vi "svl_Init Arrays for Exp Avg.vi"(0 "scaled signals":waveform(dbl)[](array[waveform]), 11 "error in (no error)":errorcluster) -> (4 "scaled signals":waveform(dbl)[](array[waveform]), 8 "initial values (impulse)":dbl[](array[numeric]) format="%.2f", 10 "dt":dbl, 14 "initial values (exp)":dbl[](array[numeric]) format="%.2f", 15 "error out":errorcluster)   [LabVIEW 2017]
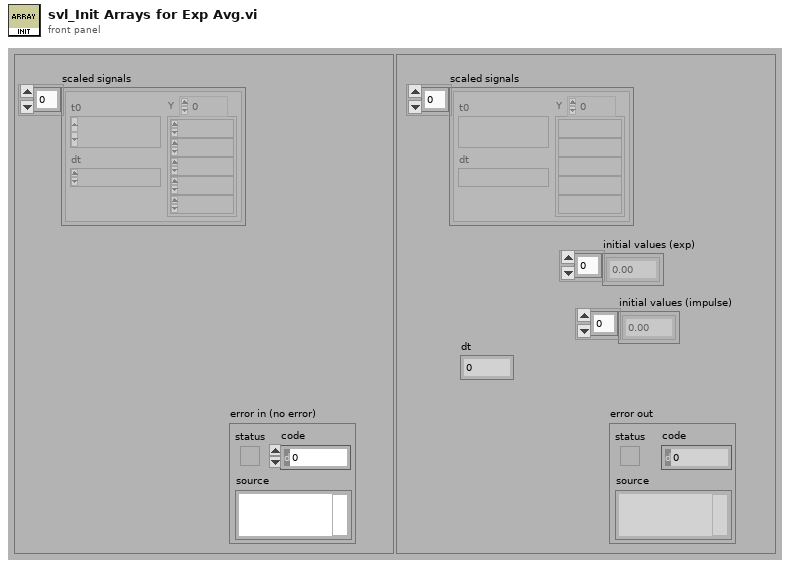
[diagram p1: front panel]
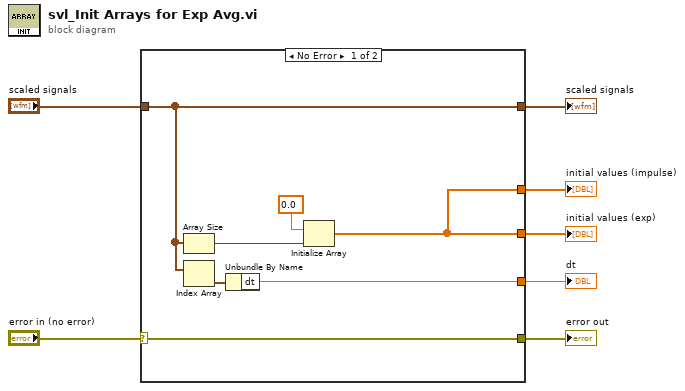
[diagram p0: block diagram]
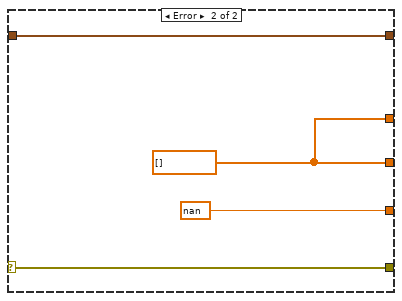
[diagram p2: hidden frame]
diagram:
  n1 = case shown="No Error" "error in (no error)" {
    selector: "error in (no error)" -> [w13 w17]
    tunnel: "scaled signals" -> [w11 w18]
    tunnel: [w8 w15] -> w7
    tunnel: [w11 w18] -> w4
    tunnel: [w13 w17] -> w3
    tunnel: [w8 w15] -> w2
    tunnel: [w9 nan ("dt")] -> w1
    frame No Error {
      n2 = Array Size(array=w11) -> (size(s)=w12:i32)
      n3 = Index Array(array=w11) -> (element=w10:waveform(dbl))  [unwired: 1 in]
      n4 = Unbundle By Name(w10) -> ("dt"=w9:dbl)
      n5 = Initialize Array(0.0 ("squaredSum"), w12) -> (w8:dbl[])
    }
    frame Error {
      w15 = dbl[] []
    }
  }
  "initial values (exp)" <- w7
  "error out" <- w3
  "scaled signals" <- w4
  "initial values (impulse)" <- w2
  "dt" <- w1
